vi "rtp play core.vi"(6 "freq":u32, 7 "rtp stop event ref":refnum<user-event>, 8 "error in (no error)":errorcluster caption="에러 입력(에러 없음)", 10 "waveform data":i8[](array[numeric]), 11 "Haptic IC 입력":refnum<class "Haptic IC.lvclass">) -> (0 "error out":errorcluster caption="에러 출력", 3 "Haptic IC 출력":refnum<class "Haptic IC.lvclass">)   [LabVIEW 2020, in "Haptic IC.lvclass"]
uses:
  Haptic IC.lvclass
  SubVIs/Serial/Controls/(Ctrl)Serial_Write Read Option.ctl
  Haptic IC.lvclass/Haptic IC.ctl
  SubVIs/Serial/Instance VIs/(SubVI)Serial_Write.vi
  SubVIs/Serial/Instance VIs/(SubVI)Serial_Write-Read.vi
panel:
  out "End Read":u8[](array[numeric])
  out "Read Array":u8[][](array[numeric])
  out "Current Read":u8[](array[numeric])
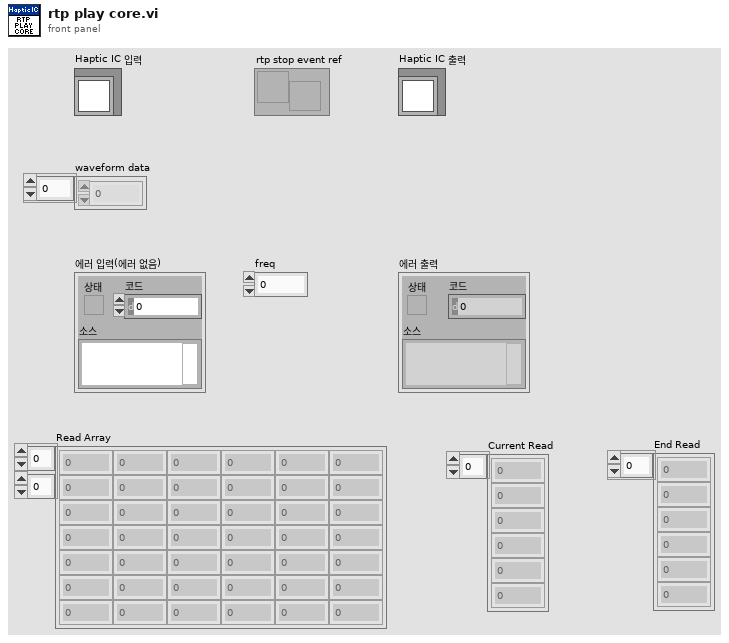
[diagram p1: front panel]
types:
  T1 = typedef "(Ctrl)Serial_Write Read Option.ctl" = cluster{"Echo Request":bool, "Header Verification":bool, "Checksum Verification":bool, "User Code Verifiaction":bool}
  T2 = typedef "Haptic IC.lvclass/(Ctrl)IC Type.ctl" = enum8{"DW7800", "DW7802", "DW7912", "DW7914"}
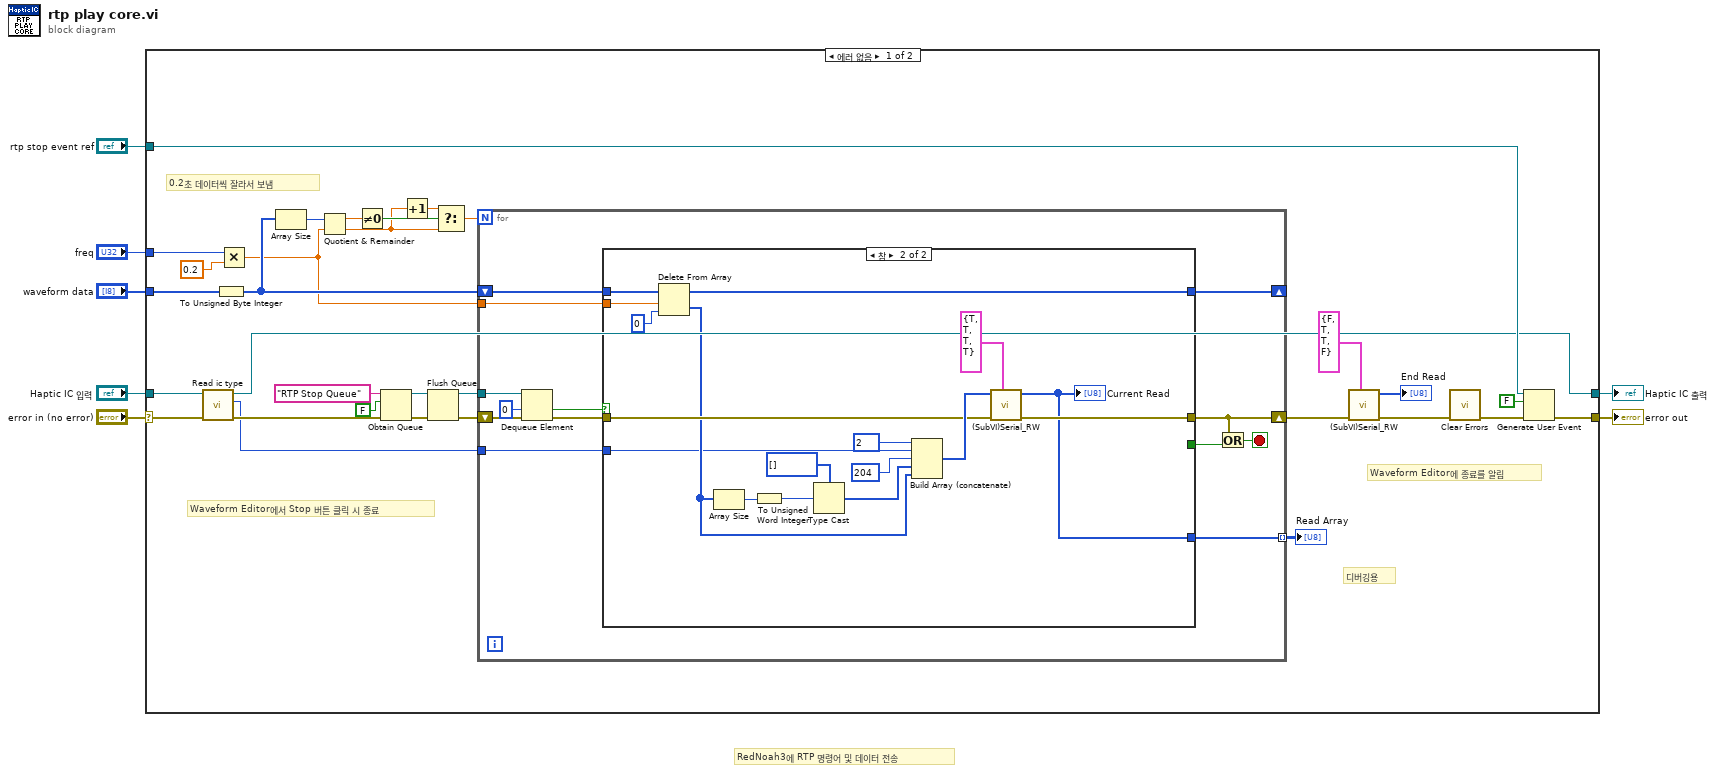
[diagram p0: block diagram]
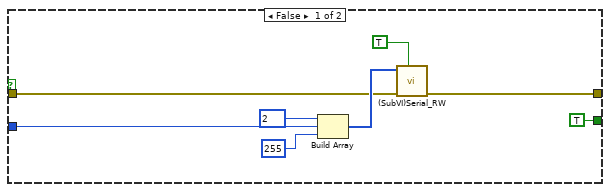
[diagram p2: hidden frame]
diagram:
  # "RedNoah3에 RTP 명령어 및 데이터 전송"
  n1 = case shown="에러 없음" "error in (no error)" {
    selector: "error in (no error)" -> [w22 w78]
    tunnel: [w11 w77] -> w6
    tunnel: "Haptic IC 입력" -> [w14 w77]
    tunnel: "freq" -> [w25 _]
    tunnel: "waveform data" -> [w24 _]
    tunnel: "rtp stop event ref" -> [w16 _]
    tunnel: [w12 w78] -> w1
    frame No Error {
      # "Waveform Editor에 종료를 알림"
      # "Waveform Editor에서 Stop 버튼 클릭 시 종료"
      # "0.2초 데이터씩 잘라서 보냄"
      # "디버깅용"
      n2 = call "Read ic type.vi"("error in (no error)"=w22, "Haptic IC 입력"=w14) -> ("error out"=w15:errorcluster, "ic type"=w13:T2, "Haptic IC 출력"=w11:refnum<class "Haptic IC.lvclass">)  [unwired: 7 in]
      n3 = To Unsigned Byte Integer(number=w24) -> (unsigned 8bit integer=w38:u8[])
      n4 = Multiply(x=w25, y=0.2) -> (x*y=w8:dbl)
      n5 = Array Size(array=w38) -> (size(s)=w37:i32)
      n6 = Quotient & Remainder(x=w37, y=w8) -> (x-y*floor(x/y)=w36:dbl, floor(x/y)=w34:dbl)
      n7 = Not Equal To 0?(x=w36) -> (x != 0?=w35:bool)
      n8 = Obtain Queue(name (unnamed)="RTP Stop Queue" ("이름(이름없음)"), element data type=FALSE, error in (no error)=w15) -> (queue out=w18:refnum<queue>, error out=w19:errorcluster)  [unwired: 2 in, 1 out]
      n9 = Increment(x=w34) -> (x+1=w33:dbl)
      n10 = Flush Queue(queue=w18, error in (no error)=w19) -> (queue out=w28:refnum<queue>, error out=w10:errorcluster)  [unwired: 1 out]
      n11 = Select(t=w33, s=w35, f=w34) -> (s? t:f=w32:dbl)
      n12 = for {
        N: w32 -> [_]
        shift-right: [w50] -> _
        shift-left: w38 -> [w51]
        tunnel: [w49] -> w31 mode=indexing
        tunnel: w8 -> [w48]
        tunnel: w28 -> [w45]
        shift-right: [w39] -> w17
        shift-left: w10 -> [w42]
        tunnel: w13 -> [w40]
        stop <- w47 stop-if-true
        n13 = Dequeue Element(queue=w45, timeout in ms (-1)=0 ("타임아웃(ms) (-1)"), error in (no error)=w42) -> (timed out?=w43:bool, error out=w41:errorcluster)  [unwired: 2 out]
        n14 = case shown="참" w43 {
          tunnel: w41 -> [w56 w69]
          tunnel: w51 -> [_ w68]
          tunnel: [_ w65] -> w50
          tunnel: [_ w61] -> w49
          tunnel: w48 -> [_ w64]
          tunnel: [w55 w62] -> w39
          tunnel: [TRUE _] -> w46
          tunnel: w40 -> [w53 w60]
          frame False {
            n15 = Build Array(u8 2, w53, u8 255) -> (w58:u8[])
            n16 = call-poly "(SubVI)Serial_RW.vi"("Echo Request"=TRUE, "error in (no error)"=w56, "Data to Write"=w58) -> ("error out"=w55:errorcluster)  [unwired: 8 in]
          }
          frame True {
            n17 = Delete From Array(array=w68, length=w64, index=0 ("인덱스")) -> (deleted portion=w66:u8[], array with subset deleted=w65:u8[])
            n18 = Array Size(array=w66) -> (size(s)=w75:i32)
            n19 = To Unsigned Word Integer(number=w75) -> (unsigned 16bit integer=w74:u16)
            n20 = Type Cast(type=u8[] [] ("타입"), x=w74) -> (*(type *) &x=w72:u8[])
            n21 = Build Array (concatenate)(u8 2, w60, u8 204, w72, w66) -> (w73:u8[])
            n22 = call-poly "(SubVI)Serial_RW.vi"("Option"=T1 {"Echo Request"=TRUE, "Header Verification"=TRUE, "Checksum Verification"=TRUE, "User Code Verifiaction"=TRUE}, "error in (no error)"=w69, "Data to Write"=w73) -> ("error out"=w62:errorcluster, "Read Data"=w61:u8[])  [unwired: 6 in, 1 out]
            "Current Read" <- w61
          }
        }
        n23 = Or(x=w39, y=w46) -> (x .or. y?=w47:bool)
      }
      "Read Array" <- w31
      n24 = call-poly "(SubVI)Serial_RW.vi"("Option"=T1 {"Echo Request"=FALSE, "Header Verification"=TRUE, "Checksum Verification"=TRUE, "User Code Verifiaction"=FALSE}, "error in (no error)"=w17) -> ("error out"=w23:errorcluster, "Read Data"=→"End Read":u8[])  [unwired: 7 in, 1 out]
      n25 = call <vilib>:"Clear Errors.vi"("error in (no error)"=w23) -> ("error out"=w27:errorcluster)  [unwired: 5 in, 1 out]
      n26 = Generate User Event(user event=w16, event data cluster=FALSE ("이벤트 데이터"), error in=w27) -> (error out=w12:errorcluster)  [unwired: 1 in, 1 out]
    }
    frame Error {
    }
  }
  "error out" <- w1
  "Haptic IC 출력" <- w6
